vi "ExtractName_ofPNGfile_fromHTML_img_src.vi"(7 "offset (0)":i32, 8 "error in (no error)":errorcluster, 10 "Identifying_String":string="img src=\"", 11 "Dencrypted HTML":string) -> (0 "error out":errorcluster, 1 "AllText":string, 2 "Found?":bool, 3 "PNG_fileName":string, 4 "FolderName":string, 5 "offset past match":i32)   [LabVIEW 2016]
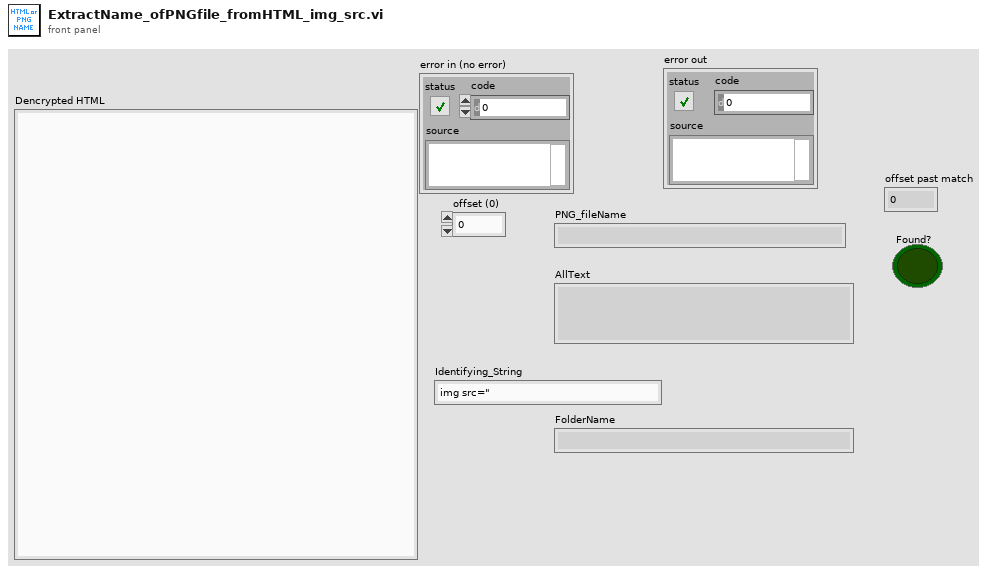
[diagram p1: front panel]
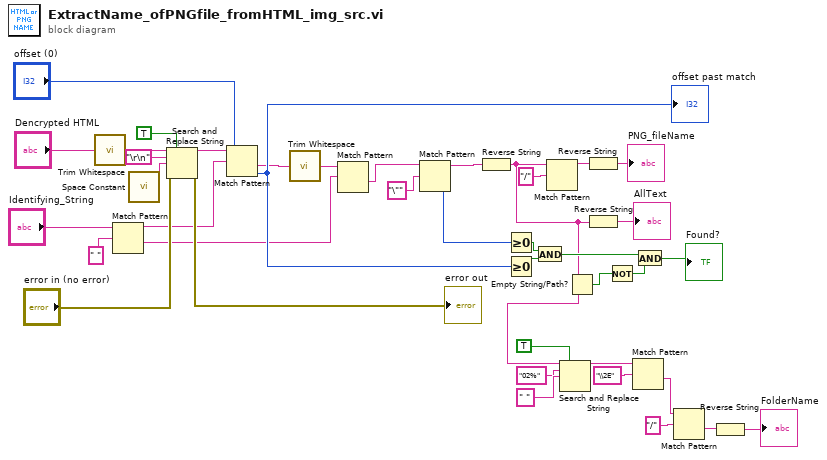
[diagram p0: block diagram]
diagram:
  n1 = call <vilib>:"Trim Whitespace.vi"("string"="Dencrypted HTML") -> ("trimmed string"=w33:string)  [unwired: 1 in]
  n2 = Match Pattern(string="Identifying_String", regular expression=" " ("search string")) -> (before substring=w16:string, after substring=w13:string)  [unwired: 1 in, 2 out]
  n3 = call <vilib>:"Space Constant.vi"() -> ("String"=w23:string)
  n4 = Search and Replace String(replace all?=TRUE ("replace all? (F)"), input string=w33, search string="\r\n", replace string=w23, error in="error in (no error)") -> (result string=w35:string, error out=→"error out":errorcluster)  [unwired: 3 in, 2 out]
  n5 = Match Pattern(string=w35, regular expression=w16, offset (0)="offset (0)") -> (after substring=w15:string, offset past match=w28:i32)  [unwired: 2 out]
  "offset past match" <- w28
  n6 = call <vilib>:"Trim Whitespace.vi"("string"=w15) -> ("trimmed string"=w14:string)  [unwired: 1 in]
  n7 = Match Pattern(string=w14, regular expression=w13) -> (after substring=w12:string)  [unwired: 1 in, 3 out]
  n8 = Match Pattern(string=w12, regular expression="\"") -> (before substring=w6:string, offset past match=w27:i32)  [unwired: 1 in, 2 out]
  n9 = Reverse String(1:w6) -> (0:w5:string)
  n10 = Greater Or Equal To 0?(x=w27) -> (x >= 0?=w26:bool)
  n11 = Greater Or Equal To 0?(x=w28) -> (x >= 0?=w25:bool)
  n12 = And(x=w26, y=w25) -> (x .and. y?=w20:bool)
  n13 = Match Pattern(string=w5, regular expression="/") -> (before substring=w39:string)  [unwired: 1 in, 3 out]
  n14 = Search and Replace String(replace all?=TRUE ("replace all? (F)"), input string=w5, search string="02%", replace string=" " ("replace string (\"\")")) -> (result string=w11:string)  [unwired: 4 in, 3 out]
  n15 = Empty String/Path?(string/path=w5) -> (empty?=w22:bool)
  n16 = Reverse String(1:w39) -> (0:→"PNG_fileName":string)
  n17 = Reverse String(1:w5) -> (0:→"AllText":string)
  n18 = Not(x=w22) -> (.not. x?=w21:bool)
  n19 = Match Pattern(string=w11, regular expression="\\2E") -> (after substring=w3:string)  [unwired: 1 in, 3 out]
  n20 = And(x=w20, y=w21) -> (x .and. y?=→"Found?":bool)
  n21 = Match Pattern(string=w3, regular expression="/") -> (after substring=w1:string)  [unwired: 1 in, 3 out]
  n22 = Reverse String(1:w1) -> (0:→"FolderName":string)
